vi "Insert Msg Queue Element__ogtk.vi"(4 "Generate Response Notifier (F)":bool, 5 "at front (F)":bool, 6 "error in (no error)":errorcluster, 7 "ms timeout (-1)":i32=-1, 8 "message":string, 9 "msg queue":T2) -> (0 "error out":errorcluster, 1 "timed out":bool, 2 "response notifier":T1, 3 "msg queue out":T2)   [LabVIEW 2011]
doc: "Inserts an element into a message queue."
uses:
  Msg Queue RefNum__ogtk.ctl
panel:
  # "[OpenG VI Tags] ***Do Not Remove***"
  # "Insert Msg Queue Element.vi\n\nInserts an element into a message queue.\n\nPlease visit http://www.OpenG.org to learn about the\nOpen Source LabVIEW software movement.\n\nNOTICE -- YOU MUST LEAVE THIS NOTICE IN PLACE.  PER THE TERMS OF THE LICENSE BELOW, YOU MAY SUBLICENSE THIS SOFTWARE \nIN ANY WAY THAT DOES NOT CONFLICT WITH THIS LICENSE.\n\n### BSD License (http://www.opensource.org/licenses/bsd-license.php) Begin ###\n\nCopyright (c) 2002, Jim Kring <jim@jimkring.com>\n\nAll rights reserved.\n\nRedistribution and use in source and binary forms, with or without modification, are permitted provided that the following conditions are met:\n\n    * Redistributions of source code must retain the above copyright notice, this list of conditions and the following disclaimer.\n    * Redistributions in binary form must reproduce the above copyright notice, this list of conditions and the following disclaimer in the \n       documentation and/or other materials provided with the distribution.\n    * Neither the name of SciWare, James Kring, Inc., nor the names of its contributors may be used to endorse or promote products derived \n       from this software without specific prior written permission.\n\nTHIS SOFTWARE IS PROVIDED BY THE COPYRIGHT HOLDERS AND CONTRIBUTORS \"AS IS\" AND ANY EXPRESS OR IMPLIED WARRANTIES, \nINCLUDING, BUT NOT LIMITED TO, THE IMPLIED WARRANTIES OF MERCHANTABILITY AND FITNESS FOR A PARTICULAR PURPOSE ARE \nDISCLAIMED. IN NO EVENT SHALL THE COPYRIGHT OWNER OR CONTRIBUTORS BE LIABLE FOR ANY DIRECT, INDIRECT, INCIDENTAL,\n SPECIAL, EXEMPLARY, OR CONSEQUENTIAL DAMAGES (INCLUDING, BUT NOT LIMITED TO, PROCUREMENT OF SUBSTITUTE GOODS OR \nSERVICES; LOSS OF USE, DATA, OR PROFITS; OR BUSINESS INTERRUPTION) HOWEVER CAUSED AND ON ANY THEORY OF LIABILITY, \nWHETHER IN CONTRACT, STRICT LIABILITY, OR TORT (INCLUDING NEGLIGENCE OR OTHERWISE) ARISING IN ANY WAY OUT OF THE USE \nOF THIS SOFTWARE, EVEN IF ADVISED OF THE POSSIBILITY OF SUCH DAMAGE.\n\n### BSD License End ###"
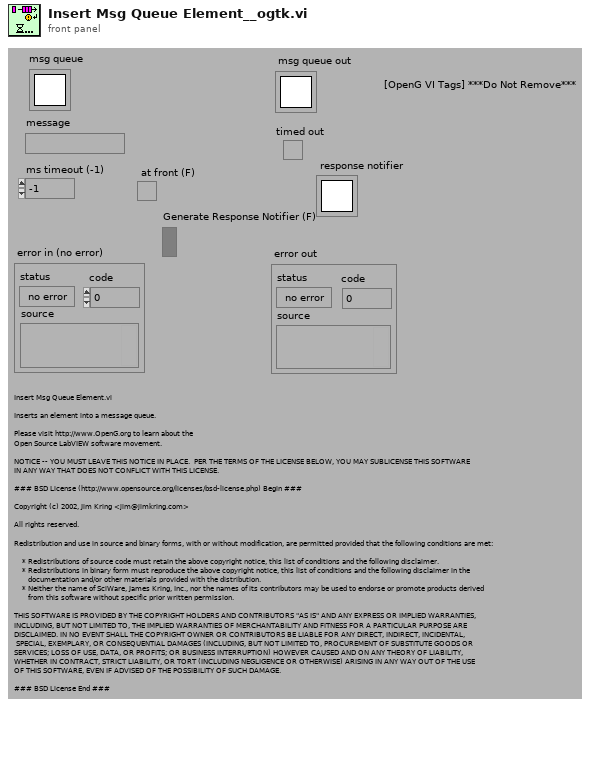
[diagram p1: front panel]
types:
  T1 = typedef "Notifier RefNum" = refnum<k1>
  T2 = typedef "Msg Queue RefNum__ogtk.ctl" = refnum<k1>
  T3 = typedef "Msg Cluster__ogtk.ctl" = cluster{"message":string, "response notifier":T1}
  T4 = typedef "Queue RefNum" = refnum<k1>
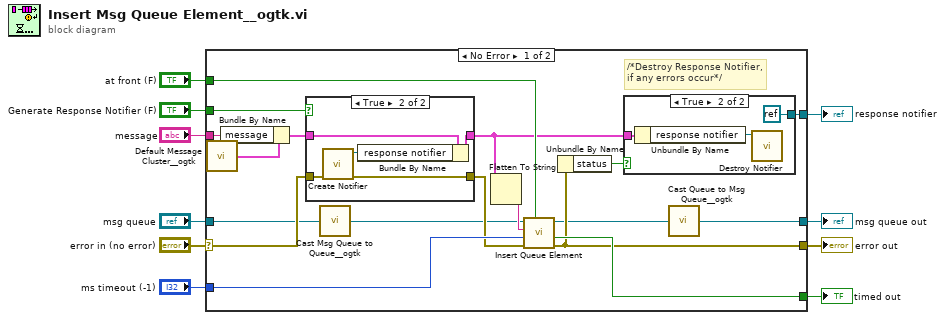
[diagram p0: block diagram]
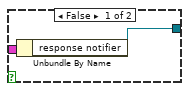
[diagram p2: hidden frame]
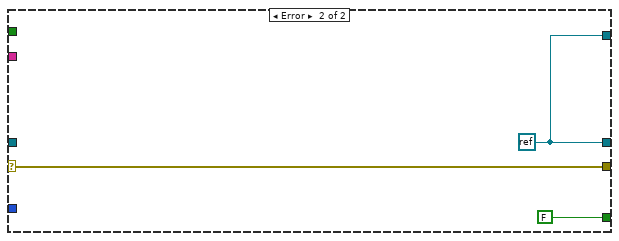
[diagram p4: hidden frame]
diagram:
  n1 = case shown="No Error" "error in (no error)" {
    selector: "error in (no error)" -> [w17 w43]
    tunnel: "at front (F)" -> [w28 _]
    tunnel: "ms timeout (-1)" -> [w27 _]
    tunnel: [w13 w41] -> w1
    tunnel: [w26 FALSE ("timed out")] -> w8
    tunnel: "message" -> [w25 _]
    tunnel: "Generate Response Notifier (F)" -> [w23 _]
    tunnel: [w18 w43] -> w5
    tunnel: [w16 w41] -> w3
    tunnel: "msg queue" -> [w11 _]
    frame No Error {
      # "/*Destroy Response Notifier, if any errors occur*/"
      n2 = call "Default Message Cluster__ogtk.vi"() -> ("default message cluster"=w12:T3)  [unwired: 5 in]
      n3 = Bundle By Name(cluster=w12, "message"=w25) -> (w24:T3)
      n4 = case shown="True" w23 {
        tunnel: w24 -> [w35 w40]
        tunnel: [w34 w36] -> w22
        tunnel: [w35 w38] -> w19
        tunnel: w17 -> [w34 w37]
        frame False {
        }
        frame True {
          n5 = call <vilib>:"Create Notifier.vi"("error in (no error)"=w37) -> ("error out"=w36:errorcluster, "notifier out"=w39:T1)  [unwired: 4 in, 1 out]
          n6 = Bundle By Name(cluster=w40, "response notifier"=w39) -> (w38:T3)
        }
      }
      n7 = call "Cast Msg Queue to Queue__ogtk.vi"("msg queue"=w11) -> ("queue"=w15:T4)  [unwired: 4 in]
      n8 = Flatten To String(anything=w19) -> (data string=w21:string)  [unwired: 3 in, 2 out]
      n9 = call <vilib>:"Insert Queue Element.vi"("at front (F)"=w28, "error in (no error)"=w22, "ms timeout (-1)"=w27, "queue element"=w21, "queue"=w15) -> ("error out"=w18:errorcluster, "timed out"=w26:bool, "queue out"=w14:T4)  [unwired: 2 in]
      n10 = Unbundle By Name(w18) -> ("status"=w20:bool)
      n11 = case shown="True" w20 {
        tunnel: w19 -> [w30 w33]
        tunnel: [w29 refnum<k0> refnum] -> w16
        frame False {
          n12 = Unbundle By Name(w30) -> ("response notifier"=w29:T1)
        }
        frame True {
          n13 = Unbundle By Name(w33) -> ("response notifier"=w32:T1)
          n14 = call <vilib>:"Destroy Notifier.vi"("notifier"=w32) -> ()  [unwired: 4 in, 3 out]
        }
      }
      n15 = call "Cast Queue to Msg Queue__ogtk.vi"("queue"=w14) -> ("msg queue"=w13:T2)  [unwired: 4 in]
    }
    frame Error {
      w41 = refnum<k0> refnum
    }
  }
  "msg queue out" <- w1
  "error out" <- w5
  "timed out" <- w8
  "response notifier" <- w3
